vi "Check PWM Output Channel Settings.vi"(8 "error in":errorcluster, 9 "read channel settings":T1[](array[typedef]), 10 "initial channel settings":T1[](array[typedef]), 11 "TestCase in":refnum<class "TestCase.lvclass">) -> (0 "error out":errorcluster, 3 "TestCase out":refnum<class "TestCase.lvclass">)   [LabVIEW 2020, in "Module Test.lvclass"]
uses:
  Module Test Classes/Module Test.lvclass
  Scripting/Modules/Mode Classes/Controls/pwm channel settings.ctl
  Scripting/Modules/Channel Classes/PWM Output Channel/Frequency.ctl
  <vilib>/addons/_JKI Toolkits/VI Tester/TestCase.llb/TestCase.lvclass
  Scripting/Modules/Channel Classes/PWM Output Channel/PWM Output Channel.lvclass
  Scripting/Scan Engine Scripting.lvlib
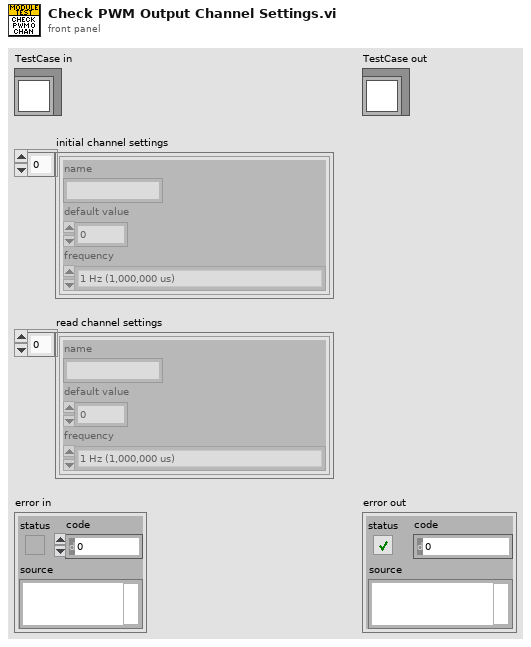
[diagram p1: front panel]
types:
  T1 = typedef "Scan Engine Scripting.lvlib/pwm channel settings.ctl" = cluster{"name":string, "default value":dbl, "frequency":T2}
  T2 = typedef "Scan Engine Scripting.lvlib/PWM Output Channel.lvclass/Frequency.ctl" = enum16{"1 Hz (1,000,000 us)", "50 Hz (20,000 us)", "250 Hz (4,000 us)", "500 Hz (2,000 us)", "1 kHz (1,000 us)", "5 kHz (200 us)", "10 kHz (100 us)", "20 kHz (50 us)"}
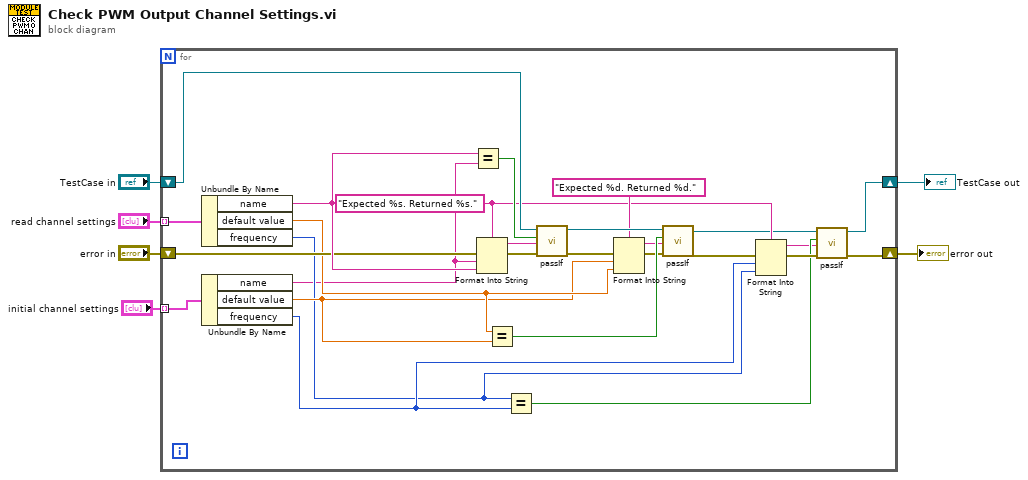
[diagram p0: block diagram]
diagram:
  n1 = for {
    tunnel: "read channel settings" -> [w32] mode=indexing
    tunnel: "initial channel settings" -> [w33] mode=indexing
    shift-right: [w8] -> w3
    shift-left: "TestCase in" -> [w31]
    shift-right: [w12] -> w1
    shift-left: "error in" -> [w28]
    w16 = "Expected %s. Returned %s." ("format string")
    n2 = Unbundle By Name(w32) -> ("name"=w29:string, "default value"=w24:dbl, "frequency"=w17:T2)
    n3 = Unbundle By Name(w33) -> ("name"=w7:string, "default value"=w21:dbl, "frequency"=w18:T2)
    n4 = Equal?(x=w29, y=w7) -> (x = y?=w30:bool)
    n5 = Format Into String(format string=w16, error in=w28, w7, w29) -> (resulting string=w9:string, error out=w27:errorcluster)  [unwired: 1 in]
    n6 = Equal?(x=w24, y=w21) -> (x = y?=w25:bool)
    n7 = Equal?(x=w17, y=w18) -> (x = y?=w14:bool)
    n8 = call-dynamic "passIf.vi"("error in (no error)"=w27, "message (\"\")"=w9, "pass"=w30, "TestCase in"=w31) -> ("error out"=w23:errorcluster, "TestCase out"=w26:refnum<class "TestCase.lvclass">)  [unwired: 6 in]
    n9 = Format Into String(format string="Expected %d. Returned %d.", error in=w23, w21, w24) -> (resulting string=w10:string, error out=w22:errorcluster)  [unwired: 1 in]
    n10 = call-dynamic "passIf.vi"("error in (no error)"=w22, "message (\"\")"=w10, "pass"=w25, "TestCase in"=w26) -> ("error out"=w15:errorcluster, "TestCase out"=w13:refnum<class "TestCase.lvclass">)  [unwired: 6 in]
    n11 = Format Into String(format string=w16, error in=w15, w18, w17) -> (resulting string=w11:string, error out=w19:errorcluster)  [unwired: 1 in]
    n12 = call-dynamic "passIf.vi"("error in (no error)"=w19, "message (\"\")"=w11, "pass"=w14, "TestCase in"=w13) -> ("error out"=w12:errorcluster, "TestCase out"=w8:refnum<class "TestCase.lvclass">)  [unwired: 6 in]
  }
  "TestCase out" <- w3
  "error out" <- w1
